vi "Alice_rapida.vi"() -> ()   [LabVIEW 2013]
uses:
  <vilib>/LabVIEW Interface for Arduino/Type Defs/Arduino Resource.ctl
  <vilib>/LabVIEW Interface for Arduino/Type Defs/Board Type.ctl
  <vilib>/LabVIEW Interface for Arduino/LabVIEW Interface for Arduino.lvlib
panel:
  out "x XOR y":string
  out "Arduino_servos":T1={"VISA resource"="", "Board Type"=enum."Uno", "Connection Type"=enum."USB / Serial", "Bytes Per Packet (15)"=15}
  in  "Alice listening port":dbl
  in  "Porta do Bob":dbl
  in  "Ip do Bob":string
  out "Bases de Bob":string
  out "Bases":string
  out "Bits enviados":string
  out "Iteração":i32=9
  in  "Nbits":dbl=20.0
  out "Base":string="r"
  out "Bit":string="0"
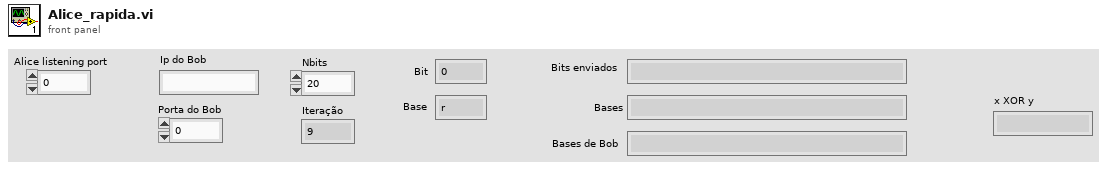
[diagram p1: front panel]
types:
  T1 = typedef "LabVIEW Interface for Arduino.lvlib/Arduino Resource.ctl" = cluster{"VISA resource":refnum<visa-resource-name>, "Board Type":T2, "Connection Type":enum8{"USB / Serial"}, "Bytes Per Packet (15)":u8}
  T2 = typedef "LabVIEW Interface for Arduino.lvlib/Board Type.ctl" = enum16{"Uno", "Dimuelanove w/Atmega 328", "Mega 2560"}
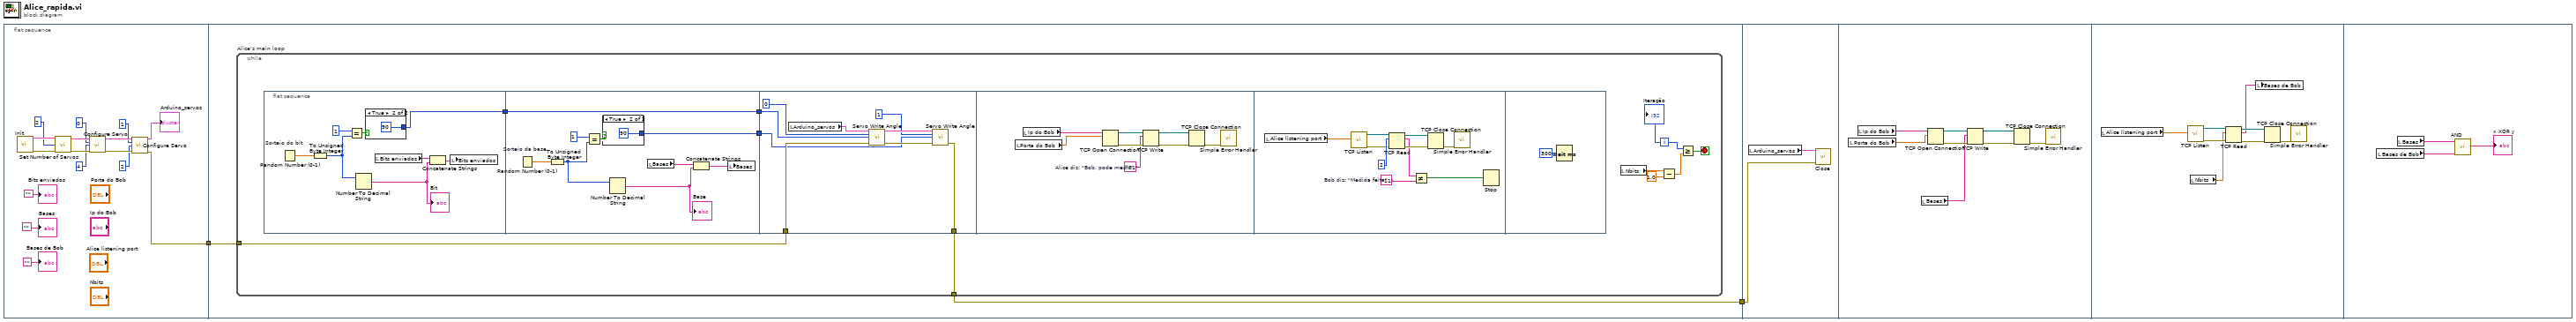
[diagram p0: block diagram]
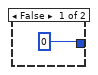
[diagram p2: hidden frame]
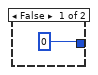
[diagram p3: hidden frame]
diagram:
  n1 = flat-sequence {
    tunnel: [w7] -> w2
    tunnel: w2 -> [w20]
    tunnel: [w19] -> w1
    tunnel: w1 -> [w81]
    frame #0 {
      n2 = call <vilib>:"Init.vi"() -> ("Arduino Resource"=w18:T1, "error out"=w17:errorcluster)  [unwired: 18 in]
      n3 = call <vilib>:"Set Number of Servos.vi"("Arduino Resource"=w18, "Number Of Servos (1)"=u8 2, "error in"=w17) -> ("Arduino Resource"=w15:T1, "error out"=w14:errorcluster)  [unwired: 11 in]
      n4 = call <vilib>:"Configure Servo.vi"("Arduino Resource"=w15, "Servo Number (0)"=u8 0, "DIO Pin (2)"=u8 4, "error in"=w14) -> ("Arduino Resource"=w13:T1, "error out"=w12:errorcluster)  [unwired: 10 in]
      n5 = call <vilib>:"Configure Servo.vi"("Arduino Resource"=w13, "Servo Number (0)"=u8 1, "DIO Pin (2)"=u8 2, "error in"=w12) -> ("Arduino Resource"=→"Arduino_servos":T1, "error out"=w7:errorcluster)  [unwired: 10 in]
      "Bits enviados" <- ""
      "Bases" <- ""
      "Bases de Bob" <- ""
    }
    frame #1 {
      n6 = while "Alice's main loop" {
        tunnel: w20 -> [w23]
        tunnel: [w22] -> w19
        i -> [w29]
        stop <- w30 stop-if-true
        n7 = flat-sequence {
          tunnel: [w34] -> w27
          tunnel: [w46] -> w28
          tunnel: w27 -> [w45]
          tunnel: [w45] -> w26
          tunnel: w28 -> [w56]
          tunnel: w26 -> [w60]
          tunnel: w23 -> [w59]
          tunnel: [w55] -> w22
          frame #0 {
            n8 = Random Number (0-1) "Sorteio do bit"() -> (number: 0 to 1=w38:dbl)
            n9 = To Unsigned Byte Integer(number=w38) -> (unsigned 8bit integer=w35:u8)
            n10 = Equal?(x=1, y=w35) -> (x = y?=w36:bool)
            n11 = Number To Decimal String(number=w35) -> (decimal integer string=w31:string)  [unwired: 1 in]
            "Bit" <- w31
            n12 = case shown="True" w36 {
              tunnel: [0 90] -> w34
              frame False {
              }
              frame True {
              }
            }
            n13 = local read "Bits enviados"() -> (w32:string)
            n14 = Concatenate Strings(w32, w31) -> (w33:string)
            n15 = local write "Bits enviados"(w33) -> ()
          }
          frame #1 {
            n16 = Random Number (0-1) "Sorteio da base"() -> (number: 0 to 1=w47:dbl)
            n17 = To Unsigned Byte Integer(number=w47) -> (unsigned 8bit integer=w42:u8)
            n18 = Equal?(x=1, y=w42) -> (x = y?=w49:bool)
            n19 = case shown="True" w49 {
              tunnel: [0 90] -> w46
              frame False {
              }
              frame True {
              }
            }
            n20 = Number To Decimal String(number=w42) -> (decimal integer string=w41:string)  [unwired: 1 in]
            "Base" <- w41
            n21 = local read "Bases"() -> (w43:string)
            n22 = Concatenate Strings(w43, w41) -> (w44:string)
            n23 = local write "Bases"(w44) -> ()
          }
          frame #2 {
            n24 = local read "Arduino_servos"() -> (w53:T1)
            n25 = call <vilib>:"Servo Write Angle.vi"("Arduino Resource"=w53, "Servo Number"=0, "Angle (Degrees)"=w60, "error in"=w59) -> ("Arduino Resource"=w58:T1, "error out"=w57:errorcluster)  [unwired: 10 in]
            n26 = call <vilib>:"Servo Write Angle.vi"("Arduino Resource"=w58, "Servo Number"=u8 1, "Angle (Degrees)"=w56, "error in"=w57) -> ("error out"=w55:errorcluster)  [unwired: 10 in, 1 out]
          }
          frame #3 {
            w61 = "01"  # Alice diz: "Bob, pode medir"
            n27 = local read "Porta do Bob"() -> (w63:dbl)
            n28 = local read "Ip do Bob"() -> (w64:string)
            n29 = TCP Open Connection(address=w64, remote port or service name=w63) -> (connection ID=w62:refnum<k5>, error out=w68:errorcluster)  [unwired: 3 in]
            n30 = TCP Write(connection ID=w62, data in=w61, error in (no error)=w68) -> (connection ID out=w67:refnum<k5>, error out=w66:errorcluster)  [unwired: 1 in, 1 out]
            n31 = TCP Close Connection(connection ID=w67, error in (no error)=w66) -> (error out=w65:errorcluster)  [unwired: 1 in, 1 out]
            n32 = call <vilib>:"Simple Error Handler.vi"("error in (no error)"=w65) -> ()  [unwired: 4 in, 5 out]
          }
          frame #4 {
            w70 = "11"  # Bob diz: "Medida feita"
            n33 = local read "Alice listening port"() -> (w69:dbl)
            n34 = call <vilib>:"TCP Listen.vi"("port"=w69) -> ("error out"=w76:errorcluster, "connection ID"=w78:refnum<k5>)  [unwired: 6 in, 3 out]
            n35 = TCP Read(connection ID=w78, bytes to read=2, error in (no error)=w76) -> (connection ID out=w74:refnum<k5>, data out=w72:string, error out=w75:errorcluster)  [unwired: 2 in]
            n36 = Not Equal?(x=w72, y=w70) -> (x != y?=w71:bool)
            n37 = TCP Close Connection(connection ID=w74, error in (no error)=w75) -> (error out=w73:errorcluster)  [unwired: 1 in, 1 out]
            n38 = call <vilib>:"Simple Error Handler.vi"("error in (no error)"=w73) -> ()  [unwired: 4 in, 5 out]
            n39 = Stop(stop? (T)=w71) -> ()
          }
          frame #5 {
            n40 = Wait (ms)(milliseconds to wait=u32 300) -> ()  [unwired: 1 out]
          }
        }
        n41 = local read "Nbits"() -> (w21:dbl)
        n42 = Subtract(x=w21, y=1.0) -> (x-y=w24:dbl)
        n43 = Greater Or Equal?(x=w29, y=w24) -> (x >= y?=w30:bool)
        "Iteração" <- w29
      }
    }
    frame #2 {
      n44 = local read "Arduino_servos"() -> (w80:T1)
      n45 = call <vilib>:"Close.vi"("Arduino Resource"=w80, "error in"=w81) -> ()  [unwired: 13 in, 1 out]
    }
    frame #3 {
      n46 = local read "Porta do Bob"() -> (w82:dbl)
      n47 = local read "Ip do Bob"() -> (w83:string)
      n48 = local read "Bases"() -> (w84:string)
      n49 = TCP Open Connection(address=w83, remote port or service name=w82) -> (connection ID=w85:refnum<k5>, error out=w89:errorcluster)  [unwired: 3 in]
      n50 = TCP Write(connection ID=w85, data in=w84, error in (no error)=w89) -> (connection ID out=w88:refnum<k5>, error out=w87:errorcluster)  [unwired: 1 in, 1 out]
      n51 = TCP Close Connection(connection ID=w88, error in (no error)=w87) -> (error out=w86:errorcluster)  [unwired: 1 in, 1 out]
      n52 = call <vilib>:"Simple Error Handler.vi"("error in (no error)"=w86) -> ()  [unwired: 4 in, 5 out]
    }
    frame #4 {
      n53 = local read "Alice listening port"() -> (w91:dbl)
      n54 = call <vilib>:"TCP Listen.vi"("port"=w91) -> ("error out"=w96:errorcluster, "connection ID"=w97:refnum<k5>)  [unwired: 6 in, 3 out]
      n55 = local read "Nbits"() -> (w90:dbl)
      n56 = TCP Read(connection ID=w97, bytes to read=w90, error in (no error)=w96) -> (connection ID out=w94:refnum<k5>, data out=w92:string, error out=w95:errorcluster)  [unwired: 2 in]
      n57 = local write "Bases de Bob"(w92) -> ()
      n58 = TCP Close Connection(connection ID=w94, error in (no error)=w95) -> (error out=w93:errorcluster)  [unwired: 1 in, 1 out]
      n59 = call <vilib>:"Simple Error Handler.vi"("error in (no error)"=w93) -> ()  [unwired: 4 in, 5 out]
    }
    frame #5 {
      n60 = local read "Bases de Bob"() -> (w99:string)
      n61 = local read "Bases"() -> (w100:string)
      n62 = call "AND.vi"("y"=w99, "x"=w100) -> ("x XOR y"=→"x XOR y":string)  [unwired: 9 in]
    }
  }
